vi "KE622x -- Get Digital I-O Params.vi"(0 "Resource In":refnum<visa-resource-name>, 1 "Check For SCPI Errors? (T)":bool=TRUE, 11 "error in (no error)":errorcluster) -> (4 "Resource Out (dupl)":refnum<visa-resource-name>, 8 "Digital I/O Params":T1={"Limit Test Enabled?"=FALSE, "Limit Test Fail Pattern"=1, "Force Output Pattern?"=FALSE, "Force Output Pattern"=0} {"Force Output Pattern" max=15 format="%04b"; "Limit Test Fail Pattern" max=15 format="%04b"}, 15 "error out":errorcluster)   [LabVIEW 2019, in "Keithley 622x.lvlib"]
doc: "Returns the parameters for Limit Testing, a.k.a. voltage limit/compliance testing."
uses:
  Keithley 622x.lvlib
  Typedefs/KE622x -- Digital I-O Params.ctl
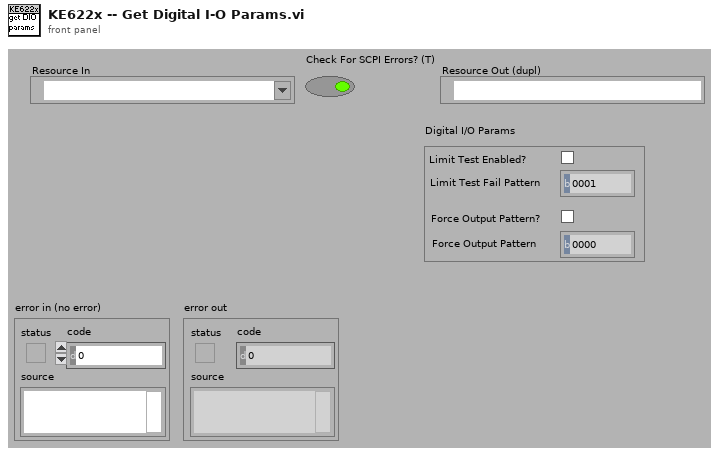
[diagram p1: front panel]
types:
  T1 = typedef "Keithley 622x.lvlib/KE622x -- Digital I-O Params.ctl" = cluster{"Limit Test Enabled?":bool, "Limit Test Fail Pattern":u8, "Force Output Pattern?":bool, "Force Output Pattern":u8}
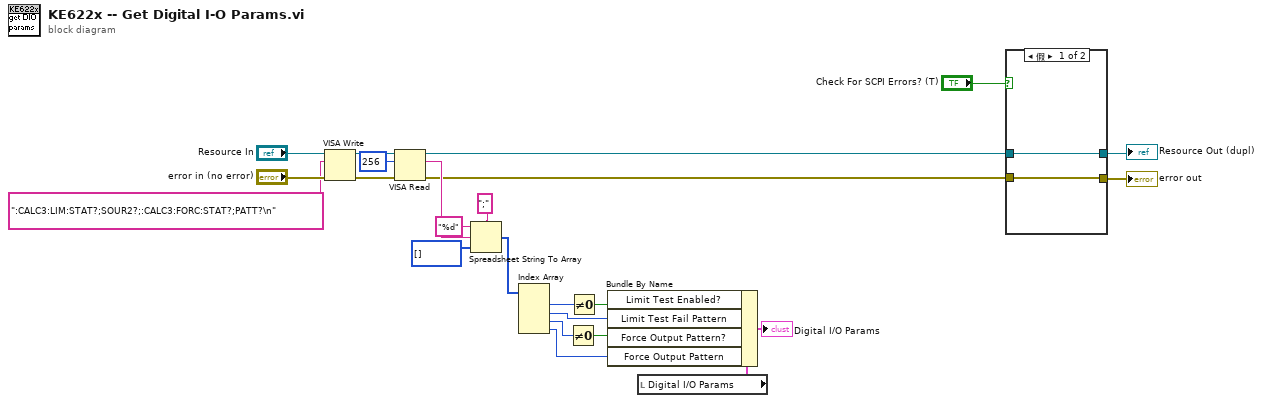
[diagram p0: block diagram]
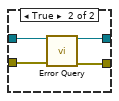
[diagram p2: hidden frame]
diagram:
  n1 = VISA Write(VISA resource name="Resource In", write buffer=":CALC3:LIM:STAT?;SOUR2?;:CALC3:FORC:STAT?;PATT?\n" ("format string"), error in (no error)="error in (no error)") -> (VISA resource name out=w18:refnum<visa-resource-name>, error out=w17:errorcluster)  [unwired: 1 out]
  n2 = VISA Read(VISA resource name=w18, byte count=u32 256, error in (no error)=w17) -> (VISA resource name out=w15:refnum<visa-resource-name>, read buffer=w14:string, error out=w8:errorcluster)  [unwired: 1 out]
  n3 = Spreadsheet String To Array(delimiter (Tab)=";", format string="%d", spreadsheet string=w14, array type (2D Dbl)=u8[] []) -> (array=w11:u8[])
  n4 = Index Array(array=w11) -> (element #1=w6:u8, element #2=w4:u8, element #3=w3:u8, element #4=w1:u8)  [unwired: 4 in]
  n5 = Not Equal To 0?(x=w3) -> (x != 0?=w2:bool)
  n6 = Not Equal To 0?(x=w6) -> (x != 0?=w5:bool)
  n7 = local read "Digital I/O Params"() -> (w10:T1)
  n8 = Bundle By Name(cluster=w10, "Limit Test Enabled?"=w5, "Limit Test Fail Pattern"=w4, "Force Output Pattern?"=w2, "Force Output Pattern"=w1) -> (→"Digital I/O Params":T1)
  n9 = case shown="假" "Check For SCPI Errors? (T)" {
    tunnel: w15 -> [w26 w30]
    tunnel: w8 -> [w25 w29]
    tunnel: [w25 w28] -> w20
    tunnel: [w26 w27] -> w21
    frame False {
    }
    frame True {
      n10 = call "Error Query.vi"("VISA Resource In"=w30, "error in (no error)"=w29) -> ("VISA Resource Out (dupl)"=w27:refnum<visa-resource-name>, "error out"=w28:errorcluster)  [unwired: 10 in, 2 out]
    }
  }
  "Resource Out (dupl)" <- w21
  "error out" <- w20
